vi "Message String FGV.vi"(6 "Action":T1, 8 "error in (no error)":errorcluster, 11 "Message String":string) -> (0 "error out":errorcluster, 3 "String out":string)   [LabVIEW 2017]
uses:
  Message String Action.ctl
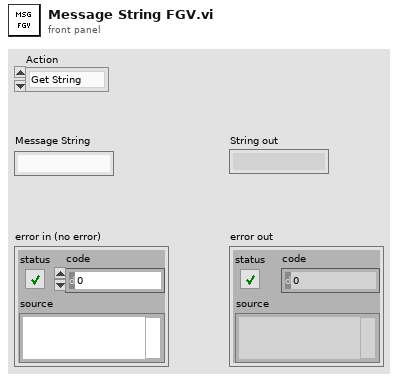
[diagram p1: front panel]
types:
  T1 = typedef "Message String Action.ctl" = enum16{"Get String", "Set String", "Reset"}
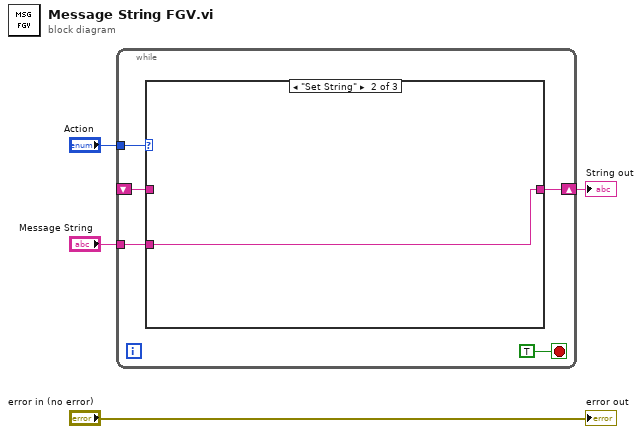
[diagram p0: block diagram]
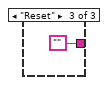
[diagram p3: hidden frame]
diagram:
  n1 = while {
    tunnel: "Action" -> [w9]
    shift-right: [w6] -> w3
    shift-left: _ -> [w7]
    tunnel: "Message String" -> [w5]
    stop <- TRUE stop-if-true
    n2 = case shown="\"Set String\"" w9 {
      tunnel: w7 -> [w10 _ _]
      tunnel: [w10 w11 ""] -> w6
      tunnel: w5 -> [_ w11 _]
      frame "Get String", Default {
      }
      frame "Set String" {
      }
      frame "Reset" {
      }
    }
  }
  "String out" <- w3
  "error out" <- "error in (no error)"
